vi "CAL GEAR TRAIN RATIO.vi"(11 "GEAR TRAIN definition":T1[](array[typedef])) -> (2 "GEAR TRAIN updated":T1[](array[typedef]), 3 "GEAR RATIO":dbl)   [LabVIEW 2023]
uses:
  ctrl defs/ctrl DEFINE GEAR.ctl
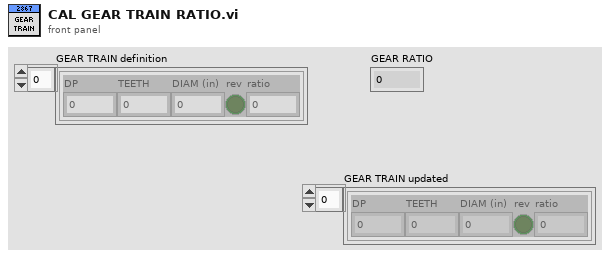
[diagram p1: front panel]
types:
  T1 = typedef "ctrl DEFINE GEAR.ctl" = cluster{"DP":dbl, "TEETH":i16, "DIAM (in)":dbl, "rev":bool, "ratio":dbl}
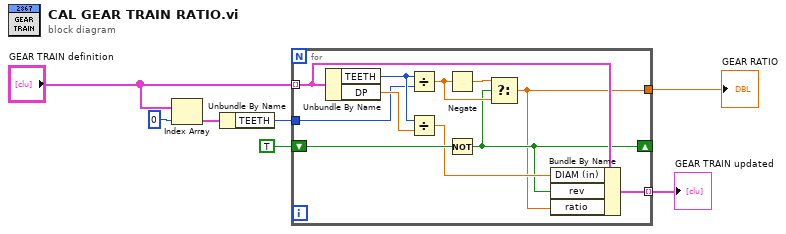
[diagram p0: block diagram]
diagram:
  n1 = Index Array(array="GEAR TRAIN definition", index=0) -> (element=w3:T1)
  n2 = Unbundle By Name(w3) -> ("TEETH"=w2:i16)
  n3 = for {
    tunnel: "GEAR TRAIN definition" -> [w18] mode=indexing
    tunnel: [w17] -> w7 mode=indexing
    shift-right: [w10] -> _
    shift-left: TRUE -> [w16]
    tunnel: w2 -> [w12]
    tunnel: [w8] -> w1
    n4 = Unbundle By Name(w18) -> ("TEETH"=w13:i16, "DP"=w14:dbl)
    n5 = Divide(x=w13, y=w12) -> (x/y=w11:dbl)
    n6 = Divide(x=w13, y=w14) -> (x/y=w15:dbl)
    n7 = Negate(x=w11) -> (-x=w9:dbl)
    n8 = Not(x=w16) -> (.not. x?=w10:bool)
    n9 = Select(t=w9, s=w10, f=w11) -> (s? t:f=w8:dbl)
    n10 = Bundle By Name(cluster=w18, "DIAM (in)"=w15, "rev"=w10, "ratio"=w8) -> (w17:T1)
  }
  "GEAR RATIO" <- w1
  "GEAR TRAIN updated" <- w7
